vi "Append Content to Page.vi"(7 "Page Content":string, 8 "error in (no error)":errorcluster {"code" format="Error %.0f"}, 10 "Page Title":string, 11 "VIDoc Printer - Confluence In":refnum<class "VIDoc Printer - Confluence.lvclass">) -> (0 "error out":errorcluster {"code" format="Error %.0f"}, 3 "VIDoc Printer - Confluence Out":refnum<class "VIDoc Printer - Confluence.lvclass">)   [LabVIEW 2023, in "VIDoc Printer - Confluence.lvlib" / "VIDoc Printer - Confluence.lvclass"]
doc: "Attempts to append <b>Page Content</b> to a page designated by <b>Page Title</b>.\n\nNo-op if no page found with <b>Page Title</b>."
uses:
  VIDoc Printer - Confluence.lvclass
  VIDoc Printer - Confluence.lvclass/VIDoc Printer - Confluence.ctl
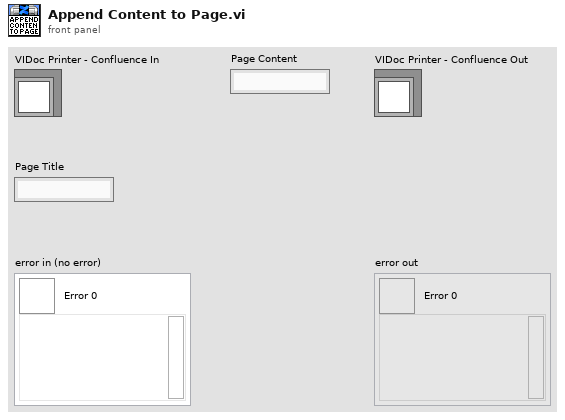
[diagram p1: front panel]
types:
  T1 = typedef "VIDoc Printer - Confluence.lvlib/VIDoc Printer - Confluence.lvclass/Page Info.ctl" = cluster{"Page":refnum<class "Page.lvclass">, "Content":string, "Attachments":set{path}}
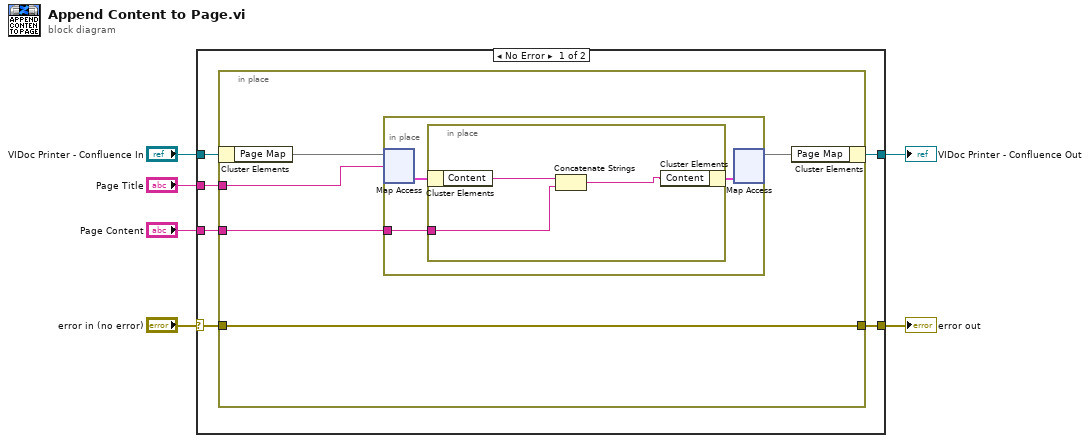
[diagram p0: block diagram]
diagram:
  n1 = case shown="No Error" "error in (no error)" {
    selector: "error in (no error)" -> [w7 w25]
    tunnel: [w8 w25] -> w5
    tunnel: [w11 w24] -> w3
    tunnel: "VIDoc Printer - Confluence In" -> [w12 w24]
    tunnel: "Page Title" -> [w10 _]
    tunnel: "Page Content" -> [w9 _]
    frame No Error {
      n2 = in-place {
        in-place-border: w10 -> [w16]
        in-place-border: w9 -> [w15]
        in-place-border: [w13] -> w8
        in-place-border: w7 -> [w13]
        n3 = in-place-cluster #1(w12) -> ("Page Map"=w17:map{string, T1})
        n4 = in-place {
          in-place-border: w15 -> [w18]
          n5 = in-place-map #2(w17, w16) -> (w20:T1)  [unwired: 1 in, 1 out]
          n6 = in-place {
            in-place-border: w18 -> [w22]
            n7 = in-place-cluster #3(w20) -> ("Content"=w23:string)
            n8 = Concatenate Strings(w23, w22) -> (w21:string)
            n9 = in-place-cluster #3("Content"=w21) -> (w19:T1)
          }
          n10 = in-place-map #2(w19) -> (w14:map{string, T1})  [unwired: 1 in, 2 out]
        }
        n11 = in-place-cluster #1("Page Map"=w14) -> (w11:refnum<class "VIDoc Printer - Confluence.lvclass">)
      }
    }
    frame Error {
    }
  }
  "error out" <- w5
  "VIDoc Printer - Confluence Out" <- w3
